vi "main.vi"() -> ()   [LabVIEW 2020]
uses:
  _controls/Notifier Cluster.ctl
  _globals/Global Controls.vi
  <resource>/objmgr/imaqdx.rc
  _controls/Global Ctrl Refs.ctl
  _controls/Trapping Laser Control.ctl
  _controls/Timer_actions.ctl
  <vilib>/userDefined/High Color/IMAQdx.ctl
  _controls/xiCam.ctl
  _controls/PCIe SLM params.ctl
  _controls/Spot Params.ctl
  _controls/PCIe SLM Spots.ctl
  _controls/PCIe SLM Zernike Coefs.ctl
  <vilib>/vision/driver/NI_Vision_Acquisition_Software.lvlib
  _controls/Exp Params.ctl
  _controls/Logging Cluster.ctl
  <vilib>/platform/TimedLoop/XDataNode/XDataNode.xnode
  <vilib>/Platform/TimedLoop/XDataNode/nitl_modes.ctl
  <vilib>/Platform/TimedLoop/XDataNode/XDNodeRunTimeDep.lvlib
  <vilib>/Platform/TimedLoop/XDataNode/wakeup.ctl
  <vilib>/Platform/TimedLoop/XDataNode/timing_clust.ctl
  _controls/SLM Real World to IMAQ Display Transform.ctl
panel:
  out "LIVE":bool
  out "ImgSat":bool
  out "xiCam":T1(plugin-control)
  out "ImgHist":u32[](graph)
  in  "Set ROI":bool
  in  "Reset ROI":bool
  out "fps":dbl caption="Camera Frame Rate (Hz)" format="%0.2f"
  out "SLM Temp (C)":dbl
  out "READY":bool
  in  "LoadXML":bool
  in  "Show Hologram":bool
  in  "SaveCurrentXML":bool
  in  "AcquireSnap":bool
  in  "stop live":bool
  in  "Cam Live Display":bool
  in  "Tab Control":T2(tab)
  in  "Camera Controls":T3={"Exposure Time (ms)"=27, "cam0 Session"="cam0", "Camera ROI"={"Width"=2048, "Height"=2048, "Offset X"=0, "Offset Y"=0}, "Command"=""} {"Camera ROI"."Offset Y" max=2046 step=2; "Camera ROI"."Offset X" max=2044 step=4; "Camera ROI"."Height" min=2 max=2048 step=2; "Camera ROI"."Width" min=4 max=2048 step=4; "Exposure Time (ms)" min=27 max=500 step=1 scale=27.0..500.0}
  in  "Spots":T5={"Spot Params"=[{"Intensity"=1.0, "Vortex"=0.0, "Phase"=0.0, "X"=0.0, "Y"=0.0, "Z"=0.0}], "Add Spot"=FALSE, "Remove Spot"=FALSE, "Clear All Spots"=FALSE, "Save Spots"=FALSE, "Generate Spots"=FALSE, "Generate Spot Pattern"=""} {"Spot Params"."Z" format="%_4g"; "Spot Params"."Y" format="%_4g"; "Spot Params"."X" format="%_4g"; "Spot Params"."Phase" format="%_4g"; "Spot Params"."Intensity" format="%_4g"}
  in  "Ventus Controls":T7 caption="Trapping Laser" {"Ventus Power" min=0.0 max=100.0 step=0.1 scale=0.0..100.0}
  in  "GridSpotsNoiseAmp":dbl=1000.0 caption="Noise Amplitude for 9x9 Grid"
  in  "Grid Size x":i32=10
  in  "Grid Size Y":i32=40
  out "Saving To Disk":i32(slide) scale=-1.0..21600.0
  out "AcqData":i32(slide) max=1000 scale=-1.0..21600.0
  in  "Exp Params":T8={"Experiment Type"="Time Series", "Experiment Name"="Experiment_1", "ExpPath"=path "D:/Data", "Save As"="TIFF", "TSFrames"=1000, "TSfps"=1.0, "Streaming"=TRUE, "tdms ref"=refnum, "frame #"=0, "Full Path"=path "", "PeakOnQueue"=FALSE} {"TSFrames" min=1 step=1; "TSfps" min=0.001 max=90.0 step=0.001 format="%_4g"}
  in  "Start Acquisition":bool
  in  "StopAcq":bool
  in  "SLM to IMAQ":T9={"Translation"={"X"=255.9856, "Y"=245.976}, "Scalling"={"xScale"=2.61758691206544, "yScale"=-2.61759}}
  out "LUT Graph":cluster{"X":dbl, "Y":dbl}[](graph)=[{"X"=-3.141592653589793, "Y"=0.0}, {"X"=-3.1169527112086968, "Y"=0.0}, {"X"=-3.0923127688276004, "Y"=0.0}, {"X"=-3.067672826446504, "Y"=0.0}, {"X"=-3.0430328840654073, "Y"=0.0}, {"X"=-3.018392941684311, "Y"=0.0}, {"X"=-2.9937529993032146, "Y"=0.0}, {"X"=-2.9691130569221182, "Y"=0.004441683995677549}, {"X"=-2.944473114541022, "Y"=0.009393597048351928}, {"X"=-2.9198331721599255, "Y"=0.014387507250025256}, {"X"=-2.8951932297788288, "Y"=0.01942901000939432}, {"X"=-2.8705532873977324, "Y"=0.024523700735155904}, {"X"=-2.845913345016636, "Y"=0.029677174836006792}, {"X"=-2.8212734026355397, "Y"=0.03489502772064378}, {"X"=-2.7966334602544434, "Y"=0.04018285479776366}, {"X"=-2.771993517873347, "Y"=0.045546251476063185}, {"X"=-2.7473535754922507, "Y"=0.050990796622549954}, {"X"=-2.722713633111154, "Y"=0.05651951641111443}, {"X"=-2.6980736907300575, "Y"=0.062130151145079436}, {"X"=-2.673433748348961, "Y"=0.06781978536195998}, {"X"=-2.648793805967865, "Y"=0.07358550359927116}, {"X"=-2.6241538635867685, "Y"=0.07942439039452798}, {"X"=-2.5995139212056717, "Y"=0.0853335302852455}, {"X"=-2.5748739788245754, "Y"=0.09131000780893878}, {"X"=-2.550234036443479, "Y"=0.09735090750312286}, {"X"=-2.5255940940623827, "Y"=0.10345331390531276}, {"X"=-2.5009541516812863, "Y"=0.10961431155302359}, {"X"=-2.47631420930019, "Y"=0.11583098498377034}, {"X"=-2.4516742669190936, "Y"=0.12210041873506809}, {"X"=-2.4270343245379973, "Y"=0.12841969734443184}, {"X"=-2.4023943821569005, "Y"=0.1347859053493767}, {"X"=-2.377754439775804, "Y"=0.14119612728741773}, {"X"=-2.353114497394708, "Y"=0.1476474476960699}, {"X"=-2.3284745550136114, "Y"=0.15413695111284825}, {"X"=-2.303834612632515, "Y"=0.16066172207526794}, {"X"=-2.2791946702514183, "Y"=0.1672188451208439}, {"X"=-2.254554727870322, "Y"=0.17380540478709125}, {"X"=-2.2299147854892256, "Y"=0.18041848561152501}, {"X"=-2.2052748431081293, "Y"=0.1870551721316602}, {"X"=-2.180634900727033, "Y"=0.19371254888501188}, {"X"=-2.1559949583459366, "Y"=0.20038770040909518}, {"X"=-2.1313550159648402, "Y"=0.20707771124142504}, {"X"=-2.106715073583744, "Y"=0.21377966591951653}, {"X"=-2.082075131202647, "Y"=0.22049064898088477}, {"X"=-2.0574351888215507, "Y"=0.22720774496304472}, {"X"=-2.0327952464404544, "Y"=0.23392803840351145}, {"X"=-2.008155304059358, "Y"=0.24064861383980002}, {"X"=-1.9835153616782615, "Y"=0.2473665558094255}, {"X"=-1.9588754192971651, "Y"=0.2540789488499029}, {"X"=-1.9342354769160686, "Y"=0.2607828774987472}, {"X"=-1.9095955345349722, "Y"=0.2674754262934736}, {"X"=-1.8849555921538759, "Y"=0.27415367977159705}, {"X"=-1.8603156497727795, "Y"=0.2808147224706326}, {"X"=-1.835675707391683, "Y"=0.2874556389280954}, {"X"=-1.8110357650105866, "Y"=0.2940735136815004}, {"X"=-1.78639582262949, "Y"=0.3006654312683626}, {"X"=-1.761755880248394, "Y"=0.30722847622619714}, {"X"=-1.7371159378672973, "Y"=0.313759733092519}, {"X"=-1.712475995486201, "Y"=0.32025628640484327}, {"X"=-1.6878360531051044, "Y"=0.326715220700685}, {"X"=-1.663196110724008, "Y"=0.3331336205175592}, {"X"=-1.6385561683429117, "Y"=0.339508570392981}, {"X"=-1.6139162259618154, "Y"=0.34583715486446537}, {"X"=-1.5892762835807188, "Y"=0.3521164584695273}, {"X"=-1.5646363411996225, "Y"=0.35834356574568205}, {"X"=-1.5399963988185261, "Y"=0.36451556123044443}, {"X"=-1.5153564564374296, "Y"=0.37062952946132965}, {"X"=-1.4907165140563332, "Y"=0.3766825549758526}, {"X"=-1.4660765716752369, "Y"=0.38267172231152863}, {"X"=-1.4414366292941405, "Y"=0.3885943072376766}, {"X"=-1.4167966869130437, "Y"=0.3944495212813968}, {"X"=-1.3921567445319474, "Y"=0.40023770070543735}, {"X"=-1.3675168021508513, "Y"=0.40595919565461763}, {"X"=-1.342876859769755, "Y"=0.41161435627375703}, {"X"=-1.3182369173886581, "Y"=0.4172035327076747}, {"X"=-1.2935969750075618, "Y"=0.42272707510119023}, {"X"=-1.2689570326264654, "Y"=0.4281853335991228}, {"X"=-1.244317090245369, "Y"=0.43357865834629183}, {"X"=-1.2196771478642725, "Y"=0.4389073994875166}, {"X"=-1.1950372054831762, "Y"=0.4441719071676165}, {"X"=-1.1703972631020798, "Y"=0.4493725315314109}, {"X"=-1.1457573207209835, "Y"=0.4545096227237191}, {"X"=-1.121117378339887, "Y"=0.45958353088936044}, {"X"=-1.0964774359587905, "Y"=0.4645946061731544}, {"X"=-1.0718374935776942, "Y"=0.4695431987199201}, {"X"=-1.0471975511965979, "Y"=0.474429658674477}, {"X"=-1.022557608815501, "Y"=0.4792543361816445}, {"X"=-0.9979176664344047, "Y"=0.48401758138624185}, {"X"=-0.9732777240533084, "Y"=0.4887197444330884}, {"X"=-0.948637781672212, "Y"=0.49336117546700364}, {"X"=-0.9239978392911157, "Y"=0.49794222463280674}, {"X"=-0.8993578969100193, "Y"=0.502463242075317}, {"X"=-0.874717954528923, "Y"=0.5069245779393541}, {"X"=-0.8500780121478266, "Y"=0.511326582369737}, {"X"=-0.8254380697667298, "Y"=0.5156696055112853}, {"X"=-0.8007981273856335, "Y"=0.5199539975088181}, {"X"=-0.7761581850045371, "Y"=0.5241801085071551}, {"X"=-0.7515182426234408, "Y"=0.5283482886511154}, {"X"=-0.726878300242344, "Y"=0.5324588880855183}, {"X"=-0.7022383578612477, "Y"=0.5365122569551832}, {"X"=-0.6775984154801513, "Y"=0.5405087454049295}, {"X"=-0.652958473099055, "Y"=0.5444487035795768}, {"X"=-0.6283185307179586, "Y"=0.5483324816239438}, {"X"=-0.6036785883368623, "Y"=0.5521604296828504}, {"X"=-0.5790386459557659, "Y"=0.5559328979011158}, {"X"=-0.5543987035746696, "Y"=0.5596502364235592}, {"X"=-0.5297587611935728, "Y"=0.563312795395}, {"X"=-0.5051188188124764, "Y"=0.5669209249602577}, {"X"=-0.4804788764313801, "Y"=0.5704749752641516}, {"X"=-0.45583893405028375, "Y"=0.5739752964515009}, {"X"=-0.43119899166918696, "Y"=0.5774222386671249}, {"X"=-0.4065590492880906, "Y"=0.5808161520558432}, {"X"=-0.3819191069069947, "Y"=0.5841573867624752}, {"X"=-0.35727916452589836, "Y"=0.5874462929318399}, {"X"=-0.33263922214480157, "Y"=0.5906832207087569}, {"X"=-0.3079992797637052, "Y"=0.5938685202380454}, {"X"=-0.2833593373826089, "Y"=0.5970025416645248}, {"X"=-0.25871939500151253, "Y"=0.6000856351330144}, {"X"=-0.23407945262041574, "Y"=0.6031181507883338}, {"X"=-0.2094395102393194, "Y"=0.606100438775302}, {"X"=-0.18479956785822305, "Y"=0.6090328492387385}, {"X"=-0.1601596254771267, "Y"=0.6119157323234626}, {"X"=-0.13551968309603035, "Y"=0.6147494381742937}, {"X"=-0.110879740714934, "Y"=0.6175343169360511}, {"X"=-0.08623979833383766, "Y"=0.6202707187535542}, {"X"=-0.06159985595274131, "Y"=0.6229589937716223}, {"X"=-0.03695991357164452, "Y"=0.6255994921350748}, {"X"=-0.012319971190548173, "Y"=0.628192563988731}, {"X"=0.012319971190548173, "Y"=0.6307385594774102}, {"X"=0.03695991357164452, "Y"=0.6332378287459319}, {"X"=0.06159985595274087, "Y"=0.6356907219391152}, {"X"=0.08623979833383721, "Y"=0.6380975892017797}, {"X"=0.110879740714934, "Y"=0.6404587806787446}, {"X"=0.13551968309603035, "Y"=0.6427746465148293}, {"X"=0.1601596254771267, "Y"=0.6450455368548531}, {"X"=0.18479956785822305, "Y"=0.6472718018436354}, {"X"=0.2094395102393194, "Y"=0.6494537916259955}, {"X"=0.23407945262041574, "Y"=0.6515918563467528}, {"X"=0.2587193950015121, "Y"=0.6536863461507265}, {"X"=0.28335933738260843, "Y"=0.6557376111827362}, {"X"=0.30799927976370567, "Y"=0.657746001587601}, {"X"=0.332639222144802, "Y"=0.6597118675101404}, {"X"=0.35727916452589836, "Y"=0.6616355590951737}, {"X"=0.3819191069069947, "Y"=0.6635174264875202}, {"X"=0.4065590492880906, "Y"=0.6653578198319992}, {"X"=0.43119899166918696, "Y"=0.6671570892734301}, {"X"=0.4558389340502833, "Y"=0.6689155849566324}, {"X"=0.48047887643137965, "Y"=0.6706336570264253}, {"X"=0.5051188188124769, "Y"=0.6723116556276281}, {"X"=0.5297587611935732, "Y"=0.6739499309050603}, {"X"=0.5543987035746696, "Y"=0.6755488330035411}, {"X"=0.5790386459557659, "Y"=0.6771087120678899}, {"X"=0.6036785883368623, "Y"=0.6786299182429261}, {"X"=0.6283185307179586, "Y"=0.6801128016734688}, {"X"=0.652958473099055, "Y"=0.6815577125043376}, {"X"=0.6775984154801513, "Y"=0.6829650008803521}, {"X"=0.7022383578612481, "Y"=0.6843350169463309}, {"X"=0.7268783002423445, "Y"=0.6856681108470939}, {"X"=0.7515182426234408, "Y"=0.6869646327274603}, {"X"=0.7761581850045371, "Y"=0.6882249327322496}, {"X"=0.8007981273856335, "Y"=0.6894493610062808}, {"X"=0.8254380697667298, "Y"=0.6906382676943738}, {"X"=0.8500780121478262, "Y"=0.6917920029413474}, {"X"=0.8747179545289221, "Y"=0.6929109168920209}, {"X"=0.8993578969100193, "Y"=0.6939953596912143}, {"X"=0.9239978392911157, "Y"=0.6950456814837462}, {"X"=0.948637781672212, "Y"=0.6960622324144364}, {"X"=0.9732777240533084, "Y"=0.6970453626281042}, {"X"=0.9979176664344047, "Y"=0.6979954222695688}, {"X"=1.022557608815501, "Y"=0.6989127614836497}, {"X"=1.0471975511965974, "Y"=0.699797730415166}, {"X"=1.0718374935776938, "Y"=0.7006506792089373}, {"X"=1.096477435958791, "Y"=0.7014719880473896}, {"X"=1.1211173783398873, "Y"=0.7022625378987619}, {"X"=1.1457573207209837, "Y"=0.703023623303892}, {"X"=1.17039726310208, "Y"=0.7037565511981412}, {"X"=1.1950372054831764, "Y"=0.7044626285168711}, {"X"=1.2196771478642727, "Y"=0.7051431621954433}, {"X"=1.244317090245369, "Y"=0.7057994591692192}, {"X"=1.2689570326264654, "Y"=0.7064328263735603}, {"X"=1.2935969750075618, "Y"=0.7070445707438283}, {"X"=1.3182369173886581, "Y"=0.7076359992153846}, {"X"=1.3428768597697545, "Y"=0.7082084187235906}, {"X"=1.3675168021508508, "Y"=0.7087631362038079}, {"X"=1.3921567445319472, "Y"=0.7093014585913984}, {"X"=1.4167966869130435, "Y"=0.7098246928217231}, {"X"=1.4414366292941398, "Y"=0.7103341458301439}, {"X"=1.4660765716752362, "Y"=0.7108311245520219}, {"X"=1.4907165140563334, "Y"=0.7113169359227188}, {"X"=1.5153564564374298, "Y"=0.7117928868775963}, {"X"=1.5399963988185261, "Y"=0.7122602843520158}, {"X"=1.5646363411996225, "Y"=0.7127204352813389}, {"X"=1.5892762835807188, "Y"=0.713174646600927}, {"X"=1.6139162259618152, "Y"=0.7136242252461416}, {"X"=1.6385561683429115, "Y"=0.7140704781523443}, {"X"=1.6631961107240079, "Y"=0.7145147122548965}, {"X"=1.687836053105105, "Y"=0.71495823448916}, {"X"=1.7124759954862014, "Y"=0.7154023517904959}, {"X"=1.7371159378672978, "Y"=0.7158483710942662}, {"X"=1.7617558802483941, "Y"=0.7162975993358321}, {"X"=1.7863958226294905, "Y"=0.7167513434505554}, {"X"=1.8110357650105868, "Y"=0.717210910373797}, {"X"=1.8356757073916832, "Y"=0.7176776070409191}, {"X"=1.8603156497727795, "Y"=0.718152740387283}, {"X"=1.8849555921538759, "Y"=0.7186376173482502}, {"X"=1.9095955345349722, "Y"=0.7191335448591821}, {"X"=1.9342354769160686, "Y"=0.7196418298554405}, {"X"=1.958875419297165, "Y"=0.7201637792723864}, {"X"=1.9835153616782613, "Y"=0.7207007000453821}, {"X"=2.0081553040593576, "Y"=0.7212538991097884}, {"X"=2.032795246440454, "Y"=0.7218246834009672}, {"X"=2.0574351888215503, "Y"=0.7224143598542799}, {"X"=2.0820751312026475, "Y"=0.7230242354050881}, {"X"=2.106715073583744, "Y"=0.7236556169887532}, {"X"=2.1313550159648402, "Y"=0.724309811540637}, {"X"=2.1559949583459366, "Y"=0.7249881259961006}, {"X"=2.180634900727033, "Y"=0.7256918672905059}, {"X"=2.2052748431081293, "Y"=0.726422342359214}, {"X"=2.2299147854892256, "Y"=0.727180858137587}, {"X"=2.254554727870322, "Y"=0.7279687215609859}, {"X"=2.279194670251419, "Y"=0.7287872395647725}, {"X"=2.3038346126325155, "Y"=0.7296377190843082}, {"X"=2.328474555013612, "Y"=0.7305214670549545}, {"X"=2.3531144973947082, "Y"=0.7314397904120732}, {"X"=2.3777544397758037, "Y"=0.7323939960910253}, {"X"=2.4023943821569, "Y"=0.7333853910271728}, {"X"=2.4270343245379964, "Y"=0.734415282155877}, {"X"=2.4516742669190927, "Y"=0.7354849764124994}, {"X"=2.47631420930019, "Y"=0.7365957807324018}, {"X"=2.5009541516812863, "Y"=0.7377490020509453}, {"X"=2.5255940940623827, "Y"=0.7389459473034917}, {"X"=2.550234036443479, "Y"=0.7401879234254024}, {"X"=2.5748739788245754, "Y"=0.7414762373520393}, {"X"=2.5995139212056717, "Y"=0.7428121960187631}, {"X"=2.624153863586768, "Y"=0.7441971063609361}, {"X"=2.6487938059678644, "Y"=0.7456322753139194}, {"X"=2.6734337483489616, "Y"=0.7471192148964195}, {"X"=2.698073690730058, "Y"=0.7486625931433437}, {"X"=2.7227136331111543, "Y"=0.7502695530679421}, {"X"=2.7473535754922507, "Y"=0.751947304031351}, {"X"=2.771993517873347, "Y"=0.7537030553947075}, {"X"=2.7966334602544434, "Y"=0.7555440165191485}, {"X"=2.8212734026355397, "Y"=0.7574773967658104}, {"X"=2.845913345016636, "Y"=0.7595104054958302}, {"X"=2.8705532873977324, "Y"=0.7616502520703445}, {"X"=2.8951932297788288, "Y"=0.7639041458504902}, {"X"=2.919833172159925, "Y"=0.7662792961974041}, {"X"=2.9444731145410215, "Y"=0.7687829124722226}, {"X"=2.969113056922118, "Y"=0.7714222040360831}, {"X"=2.993752999303214, "Y"=0.7742043802501217}, {"X"=3.0183929416843105, "Y"=0.7771366504754755}, {"X"=3.043032884065407, "Y"=0.7802262240732813}, {"X"=3.067672826446504, "Y"=0.7834803104046757}, {"X"=3.0923127688276004, "Y"=0.7869061188307955}, {"X"=3.1169527112086968, "Y"=0.7905108587127776}, {"X"=3.141592653589793, "Y"=0.7943017394117585}]
  in  "Zernikes":T10 caption="Zernike Coefficients" {"SecComaY" step=0.01; "SecComaX" step=0.01; "SecAstigY" step=0.01; "SecAstigX" step=0.01; "ComaY" step=0.01; "ComaX" step=0.01; "AstigY" step=0.01; "AstigX" step=0.01}
  in  "SLM Parameters":T11={"Width"=1920.0, "Height"=1152.0, "Board ID"=1, "Centre Y"=0.46199999999999997, "Centre X"=0.3859999999999999} {"Centre X" format="%.3g"; "Centre Y" format="%.3g"}
  in  "Master Stop":bool
  # "Notes\n\nAs of Oct 2024\n\nNon-Streaming acquisition is now controlled with the Frame Rate (Hz) control.\n\nThe slowest acquisition is 1 Hz. This is due to the limitiations of the cameras driver.\n\nPeaking during acquisition will show a real time image. Do not use in the case of high speed acquisitions as this may slow things down.\n\nSnapshots are fixed.\n\nSaving as TDMS works but is a little slower than saving as TIFF. Still advisable, since you end up with one file regardless of acquisition size."
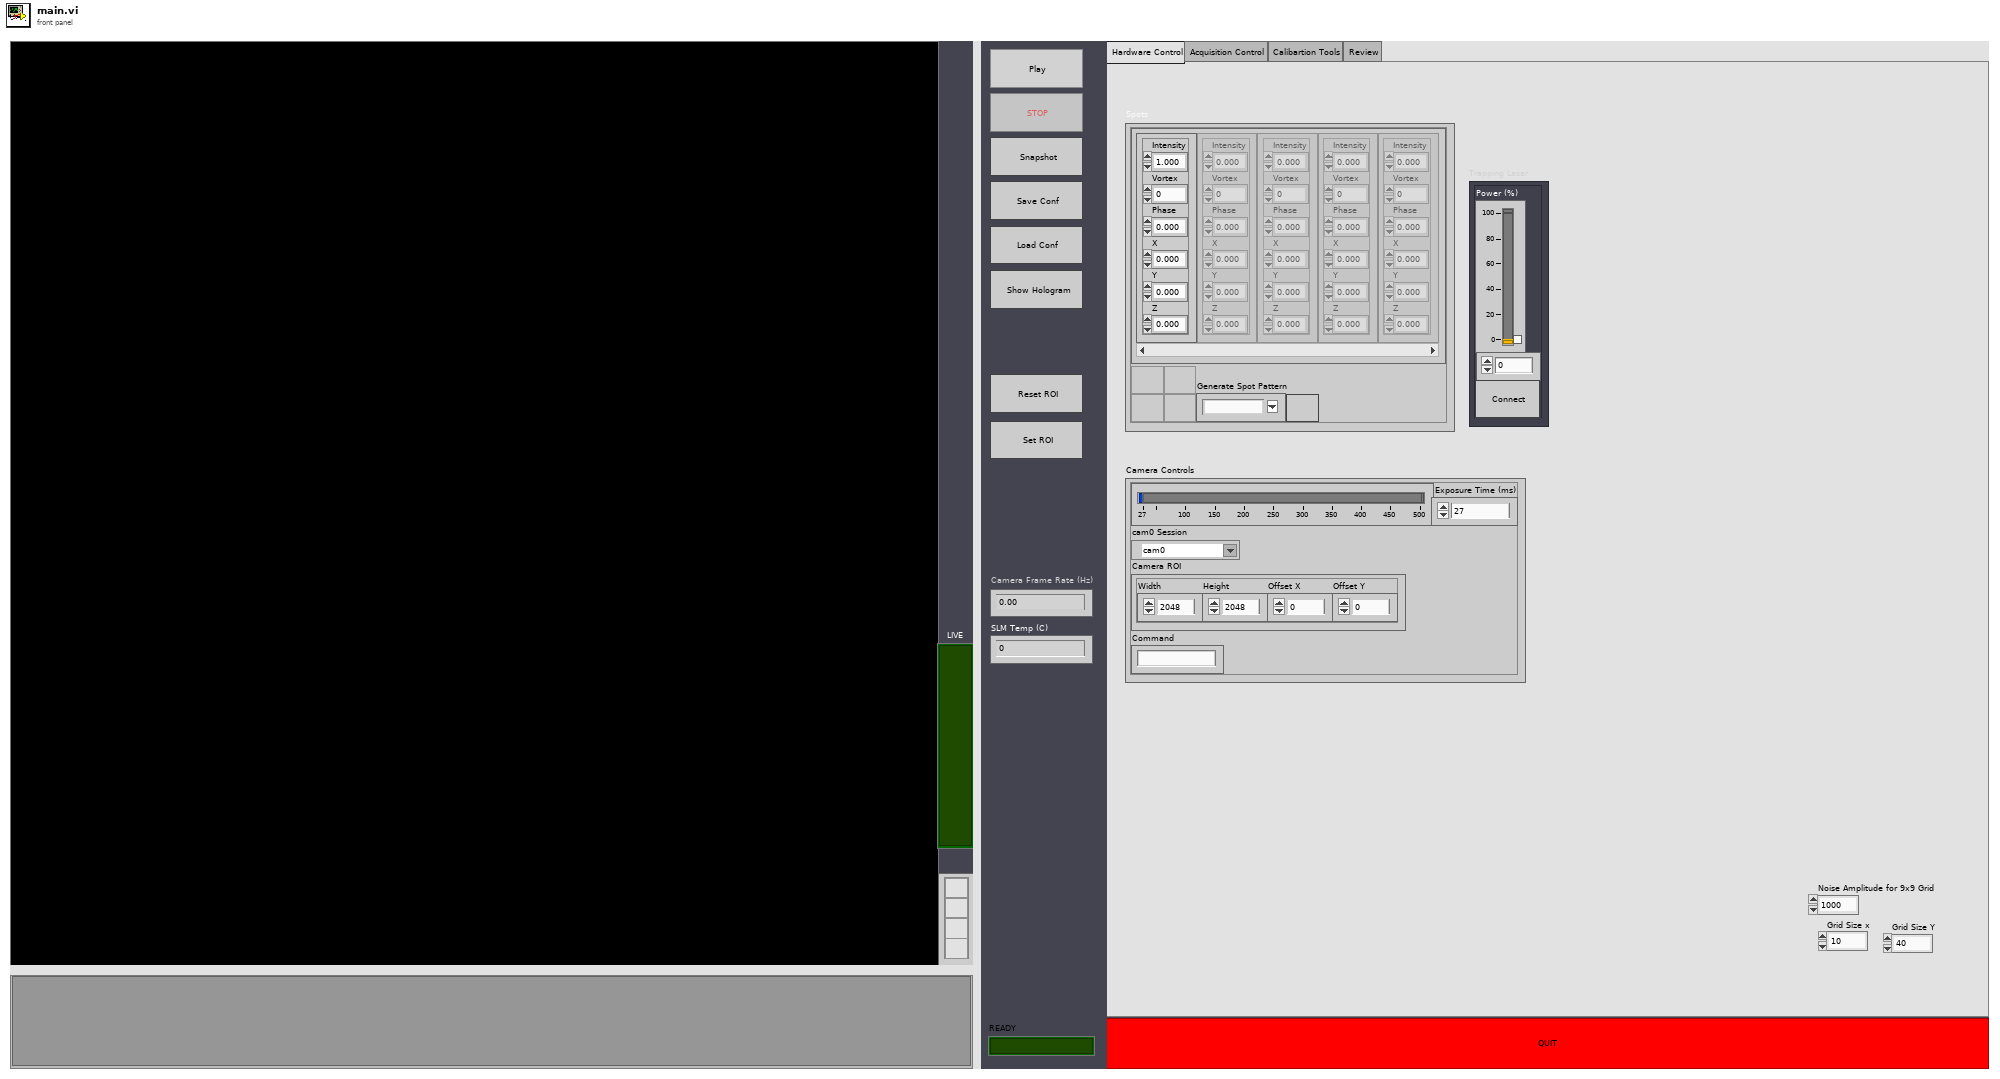
[diagram p1: front panel]
types:
  T1 = typedef "IMAQ Image.ctl" = refnum<image>
  T2 = enum32{"Hardware Control", "Acquisition Control", "Calibartion Tools", "Review"}
  T3 = typedef "xiCam.ctl" = cluster{"Exposure Time (ms)":u32, "cam0 Session":T4, "Camera ROI":cluster{"Width":u32, "Height":u32, "Offset X":u32, "Offset Y":u32}, "Command":string}
  T4 = typedef "IMAQdx.ctl" = refnum<k21>
  T5 = typedef "PCIe SLM Spots.ctl" = cluster{"Spot Params":T6, "Add Spot":bool, "Remove Spot":bool, "Clear All Spots":bool, "Save Spots":bool, "Generate Spots":bool, "Generate Spot Pattern":string}
  T6 = typedef "Spot Params.ctl" = cluster{"Intensity":dbl, "Vortex":dbl, "Phase":dbl, "X":dbl, "Y":dbl, "Z":dbl}[]
  T7 = typedef "Trapping Laser Control.ctl" = cluster{"Ventus Power":dbl, "Open Serial":bool, "VISA Refnum":refnum<visa-resource-name>}
  T8 = typedef "Exp Params.ctl" = cluster{"Experiment Type":string, "Experiment Name":string, "ExpPath":path, "Save As":string, "TSFrames":i32, "TSfps":dbl, "Streaming":bool, "tdms ref":refnum<k34>, "frame #":i64, "Full Path":path, "PeakOnQueue":bool}
  T9 = typedef "SLM Real World to IMAQ Display Transform.ctl" = cluster{"Translation":cluster{"X":dbl, "Y":dbl}, "Scalling":cluster{"xScale":dbl, "yScale":dbl}}
  T10 = typedef "PCIe SLM Zernike Coefs.ctl" = cluster{"enabled":bool, "AstigX":dbl, "AstigY":dbl, "ComaX":dbl, "ComaY":dbl, "SecAstigX":dbl, "SecAstigY":dbl, "SecComaX":dbl, "SecComaY":dbl}
  T11 = typedef "PCIe SLM params.ctl" = cluster{"Width":dbl, "Height":dbl, "Board ID":i32, "Centre Y":dbl, "Centre X":dbl}
  T12 = enum8{"Enabled", "Disabled", "Disabled and Grayed Out"}
  T13 = typedef "Image Type" = u32
  T14 = typedef "Global Ctrl Refs.ctl" = cluster{"Exp Params":refnum<vi>, "Ventus Controls":refnum<vi>, "SLM Parameters":refnum<vi>, "Spot Params":refnum<vi>, "Camera Controls":refnum<vi>}
  T15 = typedef "Global Ctrls For Saving.ctl" = cluster{"Time Stamp":cluster{"date string":string, "time string":string}, "Exp Params":T8, "Ventus Controls":T7, "Camera Controls":T3, "Spot Params":T6, "SLM Parameters":T11}
  T16 = typedef "Notifiers.ctl" = cluster{"Instrument Control":refnum<notifier>, "Live Display":refnum<notifier>, "Acquisition":refnum<notifier>}
  T17 = typedef "XDNodeRunTimeDep.lvlib/timing_clust.ctl" = cluster{"Expected End [f-1]":u64, "Actual End [f-1]":u64, "Finished Late? [f-1]":bool, "Expected End [i-1]":u64, "Actual End [i-1]":u64, "Finished Late? [i-1]":bool, "Expected Start [i]":u64, "Actual Start [i]":u64, "Expected Start [f]":u64, "Actual Start [f]":u64, "Source Name":string, "Structure Name":string, "Period":i64, "Deadline":i64, "Offset":i64, "Start":i64, "Priority":i32, "Timeout":i32, "Mode":T18, "Wakeup Reason":T19, "Error":errorcluster, "Source Type":string, "Secondary Source Type":string, "Global End Time":u64, "Global Start Time":u64, "Frame Duration":u64, "Iteration Duration":u64, "Assigned CPU":i32, "I/O Scan Engine Mode":u32}
  T18 = typedef "XDNodeRunTimeDep.lvlib/nitl_modes.ctl" = enum32{"No Change", "Process missed periods, maintain original phase", "Discard missed periods, maintain original phase", "Process missed periods, ignore original phase", "Discard missed periods, ignore original phase"}
  T19 = typedef "XDNodeRunTimeDep.lvlib/wakeup.ctl" = enum32{"Normal", "Aborted", "Asynchronous wakeup", "Timing source error", "Timed loop error", "Timeout"}
  T20 = typedef "Logging Cluster.ctl" = cluster{"Image Data Array":u8[], "Buffer Number":i32, "Timestamp (um)":u64, "Exp params":T8}
  T21 = typedef "Timer_actions.ctl" = enum16{"Reset", "Snap", "Total"}
  T22 = cluster{"Width":u32, "Height":u32, "Offset X":u32, "Offset Y":u32}
  T23 = cluster{"Exposure Time (ms)":bool, "cam0 Session":bool, "Camera ROI":cluster{"Width":bool, "Height":bool, "Offset X":bool, "Offset Y":bool}, "Command":bool}
  T24 = cluster{"Global Rectangle":i32[], "Contours":cluster{"Contour Type":u32, "ROI Type":u32, "Points":i32[]}[]}
  T25 = cluster{"Spots":T5, "SLM Parameters":T11, "Zernikes":T10}
  T26 = typedef "LVCursorListTypeDef.ctl" = cluster{"Name":string, "Color":u32, "Style":u8, "Point Style":u8, "Name Visible":bool, "Allow Drag":bool, "Cursor Mode":u32, "Plot":i32, "Index":i32, "Position":cluster{"X":dbl, "Y":dbl}, "X Scale":u32, "Y Scale":u32, "Watch Plots":i32[], "Watch All Plots":bool, "Plot Area":i32, "Label Offset":cluster{"X":dbl, "Y":dbl}}[]
  T27 = typedef "Notifier Cluster.ctl" = cluster{"message":string, "data":variant}
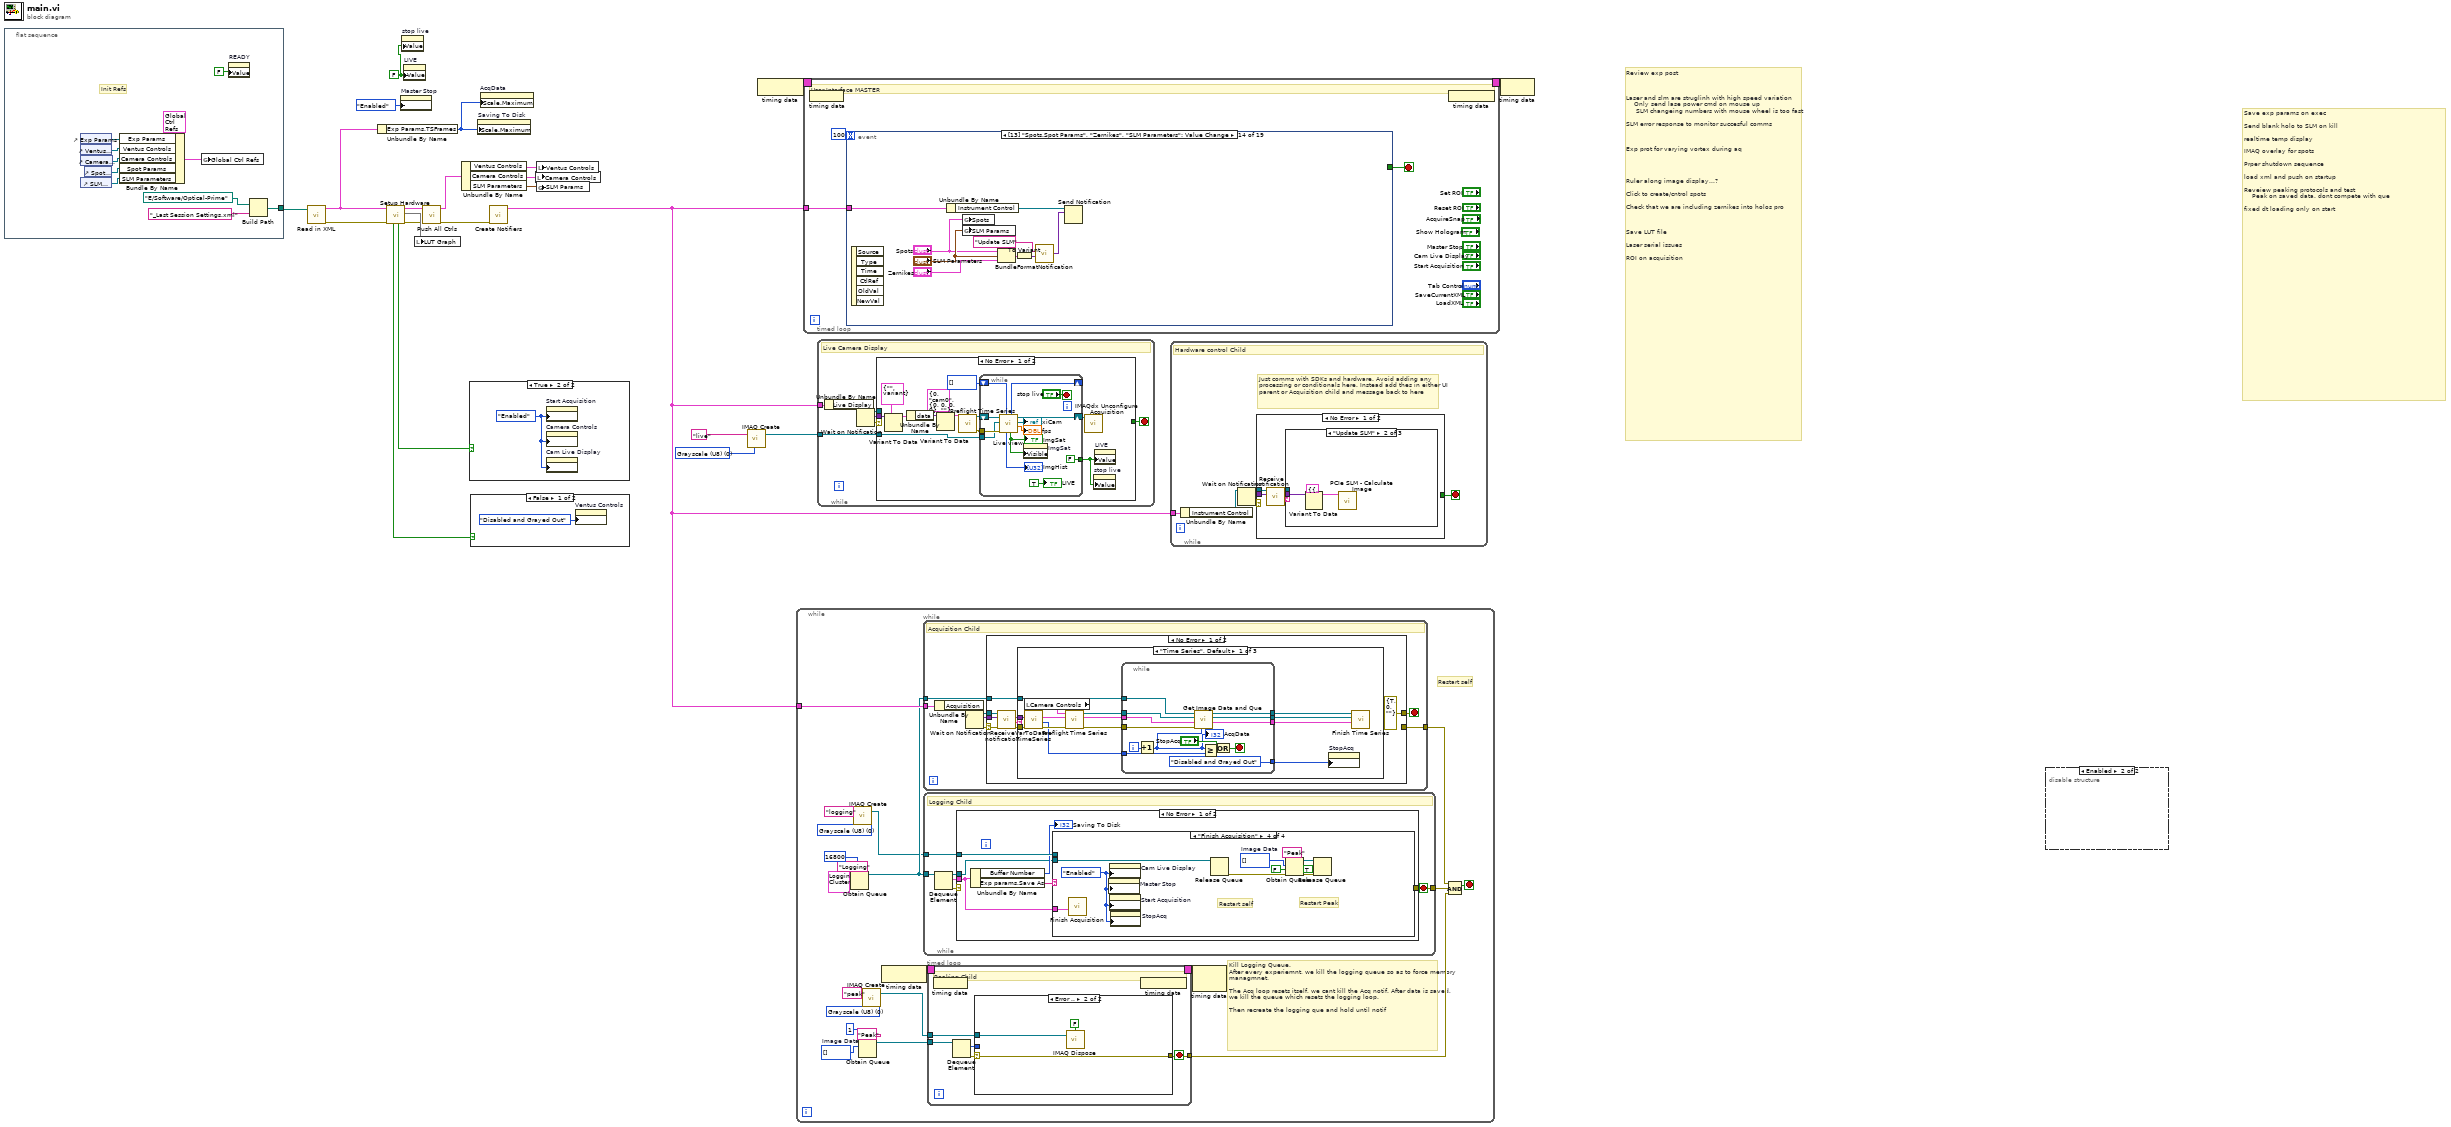
[diagram p0: block diagram]
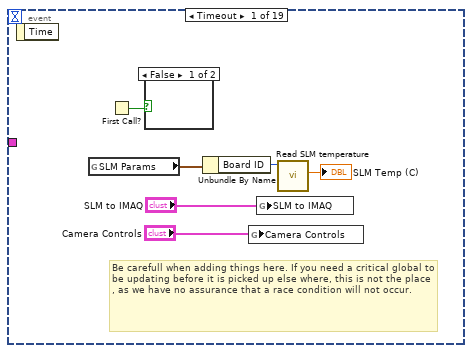
[diagram p2: hidden frame]
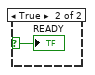
[diagram p3: hidden frame]
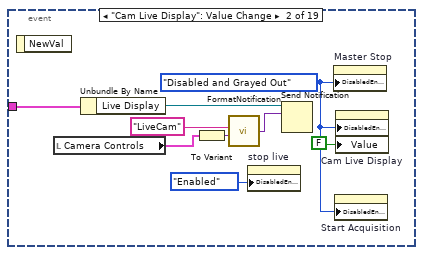
[diagram p4: hidden frame]
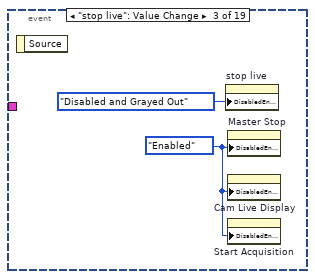
[diagram p5: hidden frame]
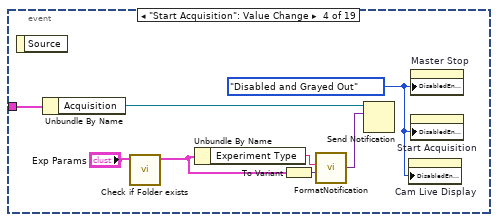
[diagram p6: hidden frame]
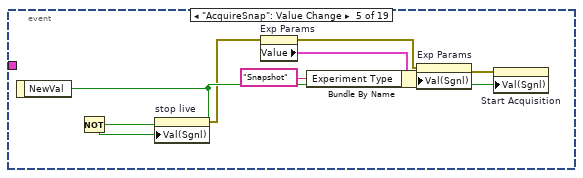
[diagram p7: hidden frame]
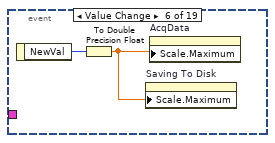
[diagram p8: hidden frame]
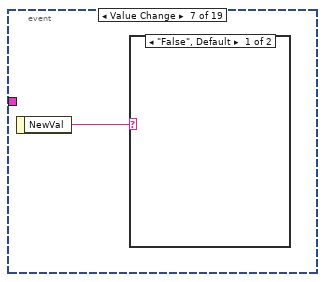
[diagram p9: hidden frame]
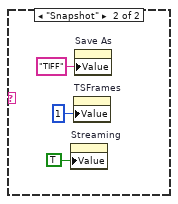
[diagram p10: hidden frame]
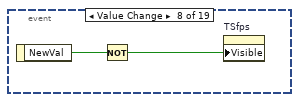
[diagram p11: hidden frame]
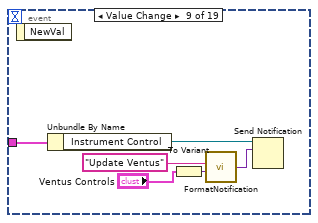
[diagram p12: hidden frame]
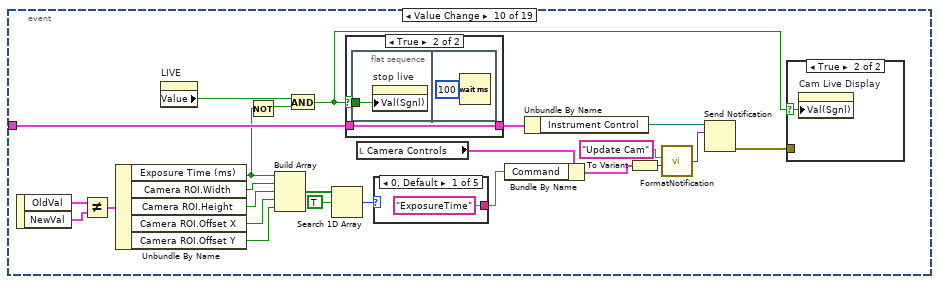
[diagram p13: hidden frame]
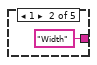
[diagram p16: hidden frame]
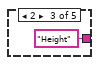
[diagram p17: hidden frame]
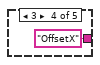
[diagram p18: hidden frame]
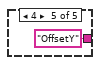
[diagram p19: hidden frame]
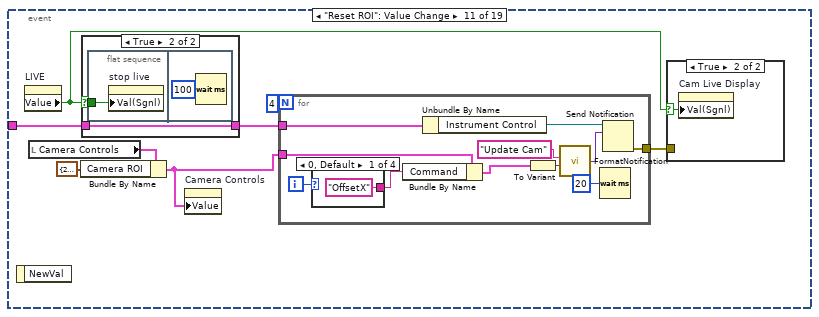
[diagram p20: hidden frame]
diagram:
  w1 = FALSE ("LIVE")
  w22 = T13 0 items=["Grayscale (U8)", "Grayscale (I16)", "Grayscale (SGL)", "Complex (CSG)", "RGB (U32)", "HSL (U32)", "RGB (U64)", "Grayscale (U16)"] ("Image Type")
  # "Save exp params on exec\n\nSend blank holo to SLM on kill\n\nrealtime temp display\n\nIMAQ overlay for spots\n\nPrper shutdown sequence\n\nload xml and push on startup\n\nReveiew peaking protocols and test\n    Peak on saved data. dont compete with que\n\nfixed dt loading only on start"
  # "Review exp post\n\n\n\nLaser and slm are struglinh with high speed variation\n    Only send lase power cmd on mouse up\n     SLM changeing numbers with mouse wheel is too fast\n\nSLM error response to monitor succesful comms\n\n\n\nExp prot for varying vortex during aq\n\n\n\n\nRuler along image display...?\n\nClick to create/cntrol spots\n\nCheck that we are including zernikes into holos pro\n\n\n\nSave LUT file\n\nLaser serial issues\n\nROI on acquisition"
  n1 = flat-sequence {
    tunnel: [w30] -> w5
    frame #0 {
      # "Init Refs"
      n2 = control-ref of="Exp Params"() -> (w27:refnum<vi>)
      n3 = control-ref of="Ventus Controls"() -> (w26:refnum<vi>)
      n4 = control-ref of="SLM Parameters"() -> (w33:refnum<vi>)
      n5 = control-ref of="Camera Controls"() -> (w23:refnum<vi>)
      n6 = control-ref of="Spot Params"() -> (w25:refnum<vi>)
      n7 = Bundle By Name(cluster=T14 {"Exp Params"=refnum, "Ventus Controls"=refnum, "SLM Parameters"=refnum, "Spot Params"=refnum, "Camera Controls"=refnum} ("Optical Prime Controls For Saving"), "Exp Params"=w27, "Ventus Controls"=w26, "Camera Controls"=w23, "Spot Params"=w25, "SLM Parameters"=w33) -> (w29:T14)
      n8 = global write "Global Controls.vi" "Global Ctrl Refs"(w29) -> ()
      n9 = property on="READY" class="Bool (strict)"("Value"=FALSE ("Boolean")) -> ()  [unwired: 2 in, 2 out]
      n10 = Build Path(base path=path "E:/Software/Optical-Prime" ("path"), name or relative path="_Last Session Settings.xml") -> (appended path=w30:path)
    }
  }
  n11 = call "Read in XML.vi"("Path to XML"=w5) -> ("error out"=w13:errorcluster, "OpticalPrime Ctrls For Saving"=w14:T15)  [unwired: 9 in]
  n12 = Unbundle By Name(w14) -> ("Exp Params.TSFrames"=w15:i32)
  n13 = call "Setup Hardware.vi"("error in (no error)"=w13, "Global Ctrls For Saving"=w14) -> ("error out"=w10:errorcluster, 2:w11, "Global Ctrls For Saving out"=w12:T15, "Camera Connected"=w17:bool, "Trapping Laser Connected"=w18:bool)  [unwired: 5 in]
  n14 = property on="Master Stop" class="Bool (strict)"("DisabledEnum"=T12."Enabled" ("Disabled")) -> ()  [unwired: 2 in, 2 out]
  n15 = property on="stop live" class="Bool (strict)"("Value"=w1) -> ()  [unwired: 2 in, 2 out]
  n16 = property on="LIVE" class="Bool (strict)"("Value"=w1) -> ()  [unwired: 2 in, 2 out]
  n17 = local write "LUT Graph"(w11) -> ()
  n18 = call "Push All Ctrls.vi"("error in"=w10, "OpticalPrime Ctrls For Saving"=w12) -> ("error out"=w7:errorcluster, "OpticalPrime Ctrls For Saving out"=w9:T15)  [unwired: 8 in]
  n19 = Unbundle By Name(w9) -> ("Ventus Controls"=w8:T7, "Camera Controls"=w4:T3, "SLM Parameters"=w6:T11)
  n20 = case shown="True" w17 {
    frame False {
      w34 = T12."Disabled and Grayed Out" ("Disabled")
      n21 = property on="Start Acquisition" class="Bool"("DisabledEnum"=w34) -> ()  [unwired: 2 in, 2 out]
      n22 = property on="Camera Controls" class="Clust (strict)"("DisabledEnum"=w34) -> ()  [unwired: 2 in, 2 out]
      n23 = property on="Cam Live Display" class="Bool (strict)"("DisabledEnum"=w34) -> ()  [unwired: 2 in, 2 out]
    }
    frame True {
      w35 = T12."Enabled" ("Disabled")
      n24 = property on="Start Acquisition" class="Bool"("DisabledEnum"=w35) -> ()  [unwired: 2 in, 2 out]
      n25 = property on="Camera Controls" class="Clust (strict)"("DisabledEnum"=w35) -> ()  [unwired: 2 in, 2 out]
      n26 = property on="Cam Live Display" class="Bool (strict)"("DisabledEnum"=w35) -> ()  [unwired: 2 in, 2 out]
    }
  }
  n27 = case shown="False" w18 {
    frame False {
      n28 = property on="Ventus Controls" class="Clust (strict)"("DisabledEnum"=T12."Disabled and Grayed Out" ("Disabled")) -> ()  [unwired: 2 in, 2 out]
    }
    frame True {
      n29 = property on="Ventus Controls" class="Clust (strict)"("DisabledEnum"=T12."Enabled" ("Disabled")) -> ()  [unwired: 2 in, 2 out]
    }
  }
  n30 = property on="Saving To Disk" class="Slide (strict)"("Scale.Maximum"=w15) -> ()  [unwired: 2 in, 2 out]
  n31 = property on="AcqData" class="Slide (strict)"("Scale.Maximum"=w15) -> ()  [unwired: 2 in, 2 out]
  n32 = call "Create Notifiers.vi"("error in (no error)"=w7) -> ("notifiers cluster"=w16:T16)  [unwired: 8 in, 2 out]
  n33 = local write "Camera Controls"(w4) -> ()
  n34 = local write "Ventus Controls"(w8) -> ()
  n35 = global write "Global Controls.vi" "SLM Params"(w6) -> ()
  n36 = call "IMAQ Create"("Image Name"="live", "Image Type"=w22) -> ("New Image"=w20:T1)  [unwired: 3 in, 1 out]
  n37 = node-c288() -> (w3:T17)
  n38 = while {
    tunnel: w16 -> [w56]
    stop <- w50 stop-if-true
    (unwired) T13 0 items=["Grayscale (U8)", "Grayscale (I16)", "Grayscale (SGL)", "Complex (CSG)", "RGB (U32)", "HSL (U32)", "RGB (U64)", "Grayscale (U16)"] ("Image Type")
    w43 = u8[] []  # Image Data
    (unwired) T13 0 items=["Grayscale (U8)", "Grayscale (I16)", "Grayscale (SGL)", "Complex (CSG)", "RGB (U32)", "HSL (U32)", "RGB (U64)", "Grayscale (U16)"] ("Image Type")
    # "Kill Logging Queue.\nAfter every experiemnt, we kill the logging queue so as to force memory managmnet.\n\nThe Acq loop resets itself, we cant kill the Acq notif. After data is saved, we kill the queue which resets the logging loop.\n\nThen recreate the logging que and hold until notif"
    # "Restart self"
    n39 = Obtain Queue(max queue size (-1, unlimited)=16800, name (unnamed)="Logging", element data type=T20 {"Image Data Array"=[], "Buffer Number"=0, "Timestamp (um)"=0, "Exp params"={"Experiment Type"="", "Experiment Name"="Experiment_1", "ExpPath"=path "D:/Data", "Save As"="TIFF", "TSFrames"=1000, "TSfps"=1.0, "Streaming"=FALSE, "tdms ref"=refnum, "frame #"=0, "Full Path"=path "", "PeakOnQueue"=FALSE}}) -> (queue out=w53:refnum<queue>)  [unwired: 2 in, 2 out]
    n40 = call "IMAQ Create"("Image Name"="logging") -> ("New Image"=w51:T1)  [unwired: 4 in, 1 out]
    n41 = Obtain Queue(max queue size (-1, unlimited)=1, name (unnamed)="Peak", element data type=w43) -> (queue out=w44:refnum<queue>)  [unwired: 2 in, 2 out]
    n42 = call "IMAQ Create"("Image Name"="peak") -> ("New Image"=w41:T1)  [unwired: 4 in, 1 out]
    n43 = node-c288() -> (w39:T17)
    n44 = while {
      tunnel: w56 -> [w110]
      tunnel: w53 -> [w105]
      tunnel: [w103] -> w48
      stop <- w104 stop-if-true
      # "Acquisition Child"
      n45 = Unbundle By Name(w110) -> ("Acquisition"=w109:refnum<notifier>)
      n46 = Wait on Notification(notifier=w109) -> (notifier out=w107:refnum<notifier>, notification=w106:variant, error out=w108:errorcluster)  [unwired: 3 in, 1 out]
      n47 = case shown="No Error" w108 {
        selector: w108 -> [w113 w165]
        tunnel: [errorcluster {"status"=TRUE, "code"=0, "source"=""} ("error IO") w165] -> w104
        tunnel: w105 -> [w115 w166]
        tunnel: w107 -> [w117 _]
        tunnel: w106 -> [w116 _]
        tunnel: [_ w165] -> w103
        frame No Error {
          n48 = call "Receive notification.vi"("error in"=w113, "Variant"=w116, "notifier in"=w117) -> ("error out"=w112:errorcluster, "message"=w114:string, "data"=w118:variant)  [unwired: 5 in, 1 out]
          n49 = case shown="\"Time Series\", Default" w114 {
            tunnel: w118 -> [w132 w160 _]
            tunnel: w115 -> [w131 w159 _]
            tunnel: w112 -> [w127 w155 _]
            frame "Time Series", Default {
              n50 = local read "Camera Controls"() -> (w128:T3)
              n51 = call "VarToData - TimeSeries.vi"("error in"=w127, "data"=w132) -> ("error out"=w126:errorcluster, "TSFrames"=w125:i32, "Exp params"=w120:T8)  [unwired: 3 in]
              n52 = call "Preflight Time Series.vi"("error in"=w126, "Exp params"=w120, "Camera Controls"=w128) -> ("error out"=w129:errorcluster, "Exp params out"=w119:T8, "CamSession out"=w130:T4)  [unwired: 6 in]
              n53 = while {
                tunnel: w129 -> [w144]
                tunnel: w125 -> [w142]
                tunnel: w119 -> [w135]
                tunnel: [w136] -> w123
                tunnel: [T12."Disabled and Grayed Out" ("Disabled")] -> w122
                tunnel: w130 -> [w146]
                tunnel: [w133] -> w121
                tunnel: w131 -> [w145]
                tunnel: [w139] -> w124
                i -> [w138]
                stop <- w140 stop-if-true
                n54 = Increment(x=w138) -> (x+1=w137:i32)
                "AcqData" <- w137
                n55 = call "Get Image Data and Que.vi"("Acquisition count"=w137, "error in (no error)"=w144, "Exp params"=w135, "Refnum in"=w146, "Queue in"=w145) -> ("Logging Cluster"=w136:T20, "Session Out"=w133:T4, "Queue out"=w139:refnum<queue>)  [unwired: 4 in]
                n56 = Greater Or Equal?(x=w137, y=w142) -> (x >= y?=w141:bool)
                n57 = Or(x="StopAcq", y=w141) -> (x .or. y?=w140:bool)
              }
              n58 = property on="StopAcq" class="Bool"("DisabledEnum"=w122) -> ()  [unwired: 2 in, 2 out]
              n59 = call "Finish Time Series.vi"("Logging Cluster"=w123, "Session In"=w121, "Queue in"=w124) -> ()  [unwired: 9 in]
            }
            frame "Snapshot" {
              n60 = call "VarToData - TimeSeries.vi"("error in"=w155, "data"=w160) -> ("error out"=w154:errorcluster, "Exp params"=w149:T8)  [unwired: 3 in, 1 out]
              n61 = local read "Camera Controls"() -> (w156:T3)
              n62 = call "Preflight Time Series.vi"("error in"=w154, "Exp params"=w149, "Camera Controls"=w156) -> ("error out"=w157:errorcluster, "Exp params out"=w148:T8, "CamSession out"=w158:T4)  [unwired: 6 in]
              n63 = call "kernelTime.vi"("Action (Snap)"=Timer_actions."Total") -> ("Microseconds"=w153:u64)  [unwired: 9 in, 1 out]
              n64 = call "Get Image Data and Que.vi"("Acquisition count"=w153, "error in (no error)"=w157, "Exp params"=w148, "Refnum in"=w158, "Queue in"=w159) -> ("Logging Cluster"=w150:T20, "Session Out"=w147:T4, "Queue out"=w151:refnum<queue>)  [unwired: 4 in]
              n65 = call "Finish Time Series.vi"("Logging Cluster"=w150, "Session In"=w147, "Queue in"=w151) -> ()  [unwired: 9 in]
            }
            frame "Dynamic Time Series" {
              # "This will be for any experiements where we want to acquire images whilst simultaneously changing another param (laser power, hologram etc).\n\nIdeally we would only be acquiring data here and sending triggers to the hardware loop."
            }
          }
        }
        frame Error {
          w164 = u8[] []  # Image Data
          # "If this errors, the notif has been destroyed so we are shutting down.\n\nKill the que, and send true to the upper loop"
          n66 = Release Queue(queue=w166) -> ()  [unwired: 2 in, 3 out]
          n67 = Obtain Queue(name (unnamed)="Peak", element data type=w164) -> (queue out=w162:refnum<queue>)  [unwired: 3 in, 2 out]
          n68 = Release Queue(queue=w162, force destroy? (F)=TRUE) -> ()  [unwired: 1 in, 3 out]
        }
      }
    }
    n69 = while {
      tunnel: w51 -> [w81]
      tunnel: w53 -> [w77]
      tunnel: [w76] -> w49
      stop <- w76 stop-if-true
      # "Logging Child"
      n70 = Dequeue Element(queue=w77) -> (queue out=w78:refnum<queue>, element=w80:T20, error out=w79:errorcluster)  [unwired: 2 in, 1 out]
      n71 = case shown="No Error" w79 {
        selector: w79 -> [_ w100]
        tunnel: w81 -> [w86 w101]
        tunnel: [_ w100] -> w76
        tunnel: w80 -> [w84 _]
        tunnel: w78 -> [w82 _]
        frame No Error {
          n72 = Unbundle By Name(w84) -> ("Buffer Number"=→"Saving To Disk":i32, "Exp params.Save As"=w83:string)
          n73 = case shown="\"Finish Acquisition\"" w83 {
            tunnel: w86 -> [w88 _ _ _]
            tunnel: w84 -> [w87 w89 _ w99]
            tunnel: w82 -> [_ _ _ w97]
            frame "TIFF", Default {
              n74 = call "Save To TIFF.vi"("Logging Cluster"=w87, "img dst"=w88) -> ()  [unwired: 9 in, 1 out]
            }
            frame "TDMS" {
              n75 = call "Save to TDMS.vi"("Logging Cluster"=w89) -> ()  [unwired: 10 in, 1 out]
            }
            frame "RAW" {
            }
            frame "Finish Acquisition" {
              w93 = u8[] []  # Image Data
              w98 = T12."Enabled" ("Disabled")
              # "Restart Peak"
              # "Restart self"
              n76 = call "Finish Acquisition.vi"("Logging Cluster"=w99) -> ()  [unwired: 11 in]
              n77 = property on="Master Stop" class="Bool (strict)"("DisabledEnum"=w98) -> ()  [unwired: 2 in, 2 out]
              n78 = property on="Cam Live Display" class="Bool (strict)"("DisabledEnum"=w98) -> ()  [unwired: 2 in, 2 out]
              n79 = property on="Start Acquisition" class="Bool"("DisabledEnum"=w98) -> ()  [unwired: 2 in, 2 out]
              n80 = property on="StopAcq" class="Bool"("DisabledEnum"=w98) -> ()  [unwired: 2 in, 2 out]
              n81 = Release Queue(queue=w97) -> (error out=w91:errorcluster)  [unwired: 2 in, 2 out]
              n82 = Obtain Queue(name (unnamed)="Peak", element data type=w93, create if not found? (T)=FALSE, error in (no error)=w91) -> (queue out=w95:refnum<queue>, error out=w90:errorcluster)  [unwired: 1 in, 1 out]
              n83 = Release Queue(queue=w95, force destroy? (F)=TRUE, error in (no error)=w90) -> ()  [unwired: 3 out]
            }
          }
        }
        frame Error {
          n84 = call "IMAQ Dispose"("All Images? (No)"=FALSE, "Image"=w101) -> ()  [unwired: 4 in, 1 out]
        }
      }
    }
    n85 = timed-loop {
      tunnel: w44 -> [w61]
      tunnel: w41 -> [w58]
      tunnel: [w57] -> w40
      timing: w39 -> [_]
      timing-out: [_] -> w38
      stop <- w57 stop-if-true
      # "Peaking Child"
      n86 = node-c288() -> ()  [unwired: 1 in]
      n87 = Dequeue Element(queue=w61) -> (element=w59:u8[], error out=w60:errorcluster)  [unwired: 2 in, 2 out]
      n88 = case shown="Error .." w60 {
        selector: w60 -> [_ w73]
        tunnel: w59 -> [w68 _]
        tunnel: w58 -> [w67 w71]
        tunnel: [_ w73] -> w57
        frame No Error {
          n89 = global read "Global Controls.vi" "Camera Controls"() -> (w66:T3)
          n90 = Unbundle By Name(w66) -> ("Camera ROI.Height"=w65:u32, "Camera ROI.Width"=w64:u32)
          n91 = Reshape Array(w68, w65, w64) -> (w69:u8[][])
          n92 = call "IMAQ ArrayToImage"("Image Pixels (U8)"=w69, "Image"=w67) -> ("Image Out"=w70:T1)  [unwired: 8 in, 1 out]
          n93 = local write "xiCam"(w70) -> ()
        }
        frame Error {
          n94 = call "IMAQ Dispose"("All Images? (No)"=FALSE, "Image"=w71) -> ()  [unwired: 4 in, 1 out]
        }
      }
      n95 = node-c288() -> ()  [unwired: 1 out]
    }
    n96 = node-c288(w38) -> ()  [unwired: 1 out]
    n97 = Compound Arithmetic op=AND(w48, w49, w40) -> (w50:bool)
  }
  n98 = timed-loop {
    tunnel: w16 -> [w167]
    timing: w3 -> [_]
    timing-out: [_] -> w2
    stop <- w169 stop-if-true
    # "User Interface MASTER"
    n99 = node-c288() -> ()  [unwired: 1 in]
    n100 = event shown="[13] \"Spots.Spot Params\", \"Zernikes\", \"SLM Parameters\": Value Change" {
      selector: _ -> [_ _ _ _ _ _ _ _ _ _ _ _ _ _ _ _ _ _ _]
      dyn-events: _ -> [_ _ _ _ _ _ _ _ _ _ _ _ _ _ _ _ _ _ _]
      timeout: 100 -> [_ _ _ _ _ _ _ _ _ _ _ _ _ _ _ _ _ _ _]
      tunnel: [_ _ _ _ _ _ _ _ _ _ _ _ _ _ _ _ _ _ TRUE] -> w169
      tunnel: w167 -> [_ w187 _ w196 _ _ _ _ w216 w227 w262 w292 _ w328 _ _ _ _ w375]
      event Timeout {
        # "Be carefull when adding things here. If you need a critical global to be updating before it is picked up else where, this is not the place , as we have no assurance that a race condition will not occur."
        n101 = event-data() -> ()  [unwired: 1 in, 1 out]
        n102 = global read "Global Controls.vi" "SLM Params"() -> (w176:T11)
        n103 = First Call?() -> (First Call?: T/F=w173:bool)
        n104 = case shown="False" w173 {
          selector: w173 -> [_ w178]
          frame False {
          }
          frame True {
            "READY" <- w178
          }
        }
        n105 = Unbundle By Name(w176) -> ("Board ID"=w177:i32)
        n106 = global write "Global Controls.vi" "Camera Controls"("Camera Controls") -> ()
        n107 = global write "Global Controls.vi" "SLM to IMAQ"("SLM to IMAQ") -> ()
        n108 = call <userlib>:"Read SLM temperature.vi"("board IN"=w177) -> ("temperature"=→"SLM Temp (C)":dbl)  [unwired: 8 in, 2 out]
      }
      event "Cam Live Display": Value Change {
        w184 = T12."Disabled and Grayed Out" ("Disabled")
        n109 = event-data() -> ()  [unwired: 1 in, 1 out]
        n110 = local read "Camera Controls"() -> (w182:T3)
        n111 = Unbundle By Name(w187) -> ("Live Display"=w186:refnum<notifier>)
        n112 = To Variant(anything=w182) -> (Variant=w183:variant)
        n113 = call "FormatNotification.vi"("Param in variant form"=w183, "message"="LiveCam") -> ("Notification"=w180:variant)  [unwired: 2 in]
        n114 = property on="stop live" class="Bool (strict)"("DisabledEnum"=T12."Enabled" ("Disabled")) -> ()  [unwired: 2 in, 2 out]
        n115 = Send Notification(notification=w180, notifier=w186) -> ()  [unwired: 1 in, 2 out]
        n116 = property on="Master Stop" class="Bool (strict)"("DisabledEnum"=w184) -> ()  [unwired: 2 in, 2 out]
        n117 = property on="Start Acquisition" class="Bool"("DisabledEnum"=w184) -> ()  [unwired: 2 in, 2 out]
        n118 = property on="Cam Live Display" class="Bool (strict)"("DisabledEnum"=w184, "Value"=FALSE ("Cam Live Display")) -> ()  [unwired: 2 in, 2 out]
      }
      event "stop live": Value Change {
        w189 = T12."Enabled" ("Disabled")
        n119 = event-data() -> ()  [unwired: 1 in, 1 out]
        n120 = property on="stop live" class="Bool (strict)"("DisabledEnum"=T12."Disabled and Grayed Out" ("Disabled")) -> ()  [unwired: 2 in, 2 out]
        n121 = property on="Master Stop" class="Bool (strict)"("DisabledEnum"=w189) -> ()  [unwired: 2 in, 2 out]
        n122 = property on="Cam Live Display" class="Bool (strict)"("DisabledEnum"=w189) -> ()  [unwired: 2 in, 2 out]
        n123 = property on="Start Acquisition" class="Bool"("DisabledEnum"=w189) -> ()  [unwired: 2 in, 2 out]
      }
      event "Start Acquisition": Value Change {
        w195 = T12."Disabled and Grayed Out" ("Disabled")
        n124 = event-data() -> ()  [unwired: 1 in, 1 out]
        n125 = Unbundle By Name(w196) -> ("Acquisition"=w197:refnum<notifier>)
        n126 = call "Check if Folder exists.vi"("Exp Params in"="Exp Params") -> ("Exp Params out"=w193:T8)  [unwired: 9 in, 1 out]
        n127 = Unbundle By Name(w193) -> ("Experiment Type"=w192:string)
        n128 = To Variant(anything=w193) -> (Variant=w194:variant)
        n129 = call "FormatNotification.vi"("Param in variant form"=w194, "message"=w192) -> ("Notification"=w191:variant)  [unwired: 2 in]
        n130 = Send Notification(notification=w191, notifier=w197) -> ()  [unwired: 1 in, 2 out]
        n131 = property on="Cam Live Display" class="Bool (strict)"("DisabledEnum"=w195) -> ()  [unwired: 2 in, 2 out]
        n132 = property on="Master Stop" class="Bool (strict)"("DisabledEnum"=w195) -> ()  [unwired: 2 in, 2 out]
        n133 = property on="Start Acquisition" class="Bool"("DisabledEnum"=w195) -> ()  [unwired: 2 in, 2 out]
      }
      event "AcquireSnap": Value Change {
        n134 = event-data() -> ("NewVal"=w201:bool)  [unwired: 1 in]
        n135 = Not(x=w201) -> (.not. x?=w200:bool)
        n136 = property on="stop live" class="Bool (strict)"("Val(Sgnl)"=w200) -> (error out=w199:errorcluster)  [unwired: 2 in, 1 out]
        n137 = property on="Exp Params" class="Clust (strict)"(error in=w199) -> (error out=w198:errorcluster, "Value"=w204:T8)  [unwired: 1 in, 1 out]
        n138 = Bundle By Name(cluster=w204, "Experiment Type"="Snapshot") -> (w205:T8)
        n139 = property on="Exp Params" class="Clust (strict)"(error in=w198, "Val(Sgnl)"=w205) -> (error out=w202:errorcluster)  [unwired: 1 in, 1 out]
        n140 = property on="Start Acquisition" class="Bool"(error in=w202, "Val(Sgnl)"=w201) -> ()  [unwired: 1 in, 2 out]
      }
      event Value Change {
        n141 = event-data() -> ("NewVal"=w207:i32)  [unwired: 1 in]
        n142 = To Double Precision Float(number=w207) -> (double precision float=w206:dbl)
        n143 = property on="Saving To Disk" class="Slide (strict)"("Scale.Maximum"=w206) -> ()  [unwired: 2 in, 2 out]
        n144 = property on="AcqData" class="Slide (strict)"("Scale.Maximum"=w206) -> ()  [unwired: 2 in, 2 out]
      }
      event Value Change {
        n145 = event-data() -> ("NewVal"=w208:string)  [unwired: 1 in]
        n146 = case shown="\"False\", Default" w208 {
          frame "False", Default {
          }
          frame "Snapshot" {
            n147 = property on="Streaming" class="Bool (strict)"("Value"=TRUE) -> ()  [unwired: 2 in, 2 out]
            n148 = property on="TSFrames" class="DigNum (strict)"("Value"=1) -> ()  [unwired: 2 in, 2 out]
            n149 = property on="Save As" class="CmbBox"("Value"="TIFF") -> ()  [unwired: 2 in, 2 out]
          }
        }
      }
      event Value Change {
        n150 = event-data() -> ("NewVal"=w213:bool)  [unwired: 1 in]
        n151 = Not(x=w213) -> (.not. x?=w212:bool)
        n152 = property on="TSfps" class="DigNum (strict)"("Visible"=w212) -> ()  [unwired: 2 in, 2 out]
      }
      event Value Change {
        n153 = event-data() -> ()  [unwired: 1 in, 1 out]
        n154 = Unbundle By Name(w216) -> ("Instrument Control"=w217:refnum<notifier>)
        n155 = To Variant(anything="Ventus Controls") -> (Variant=w215:variant)
        n156 = call "FormatNotification.vi"("Param in variant form"=w215, "message"="Update Ventus") -> ("Notification"=w218:variant)  [unwired: 2 in]
        n157 = Send Notification(notification=w218, notifier=w217) -> ()  [unwired: 1 in, 2 out]
      }
      event Value Change {
        n158 = event-data() -> ("OldVal"=w243:T3, "NewVal"=w242:T3)  [unwired: 1 in]
        n159 = Not Equal?(x=w243, y=w242) -> (x != y?=w241:T23)
        n160 = Unbundle By Name(w241) -> ("Exposure Time (ms)"=w222:bool, "Camera ROI.Width"=w240:bool, "Camera ROI.Height"=w239:bool, "Camera ROI.Offset X"=w238:bool, "Camera ROI.Offset Y"=w237:bool)
        n161 = property on="LIVE" class="Bool (strict)"() -> ("Value"=w223:bool)  [unwired: 2 in, 2 out]
        n162 = Not(x=w222) -> (.not. x?=w221:bool)
        n163 = Build Array(w222, w240, w239, w238, w237) -> (w236:bool[])
        n164 = And(x=w223, y=w221) -> (x .and. y?=w224:bool)
        n165 = Search 1D Array(1D array=w236, element=TRUE) -> (index of element=w234:i32)  [unwired: 1 in]
        n166 = case shown="True" w224 {
          selector: w224 -> [_ w246]
          tunnel: w227 -> [w245 w247]
          tunnel: [w245 w247] -> w226
          frame False {
          }
          frame True {
            n167 = flat-sequence {
              tunnel: w246 -> [w248]
              frame #0 {
                n168 = property on="stop live" class="Bool (strict)"("Val(Sgnl)"=w248) -> ()  [unwired: 2 in, 2 out]
              }
              frame #1 {
                n169 = Wait (ms)(milliseconds to wait=u32 100) -> ()  [unwired: 1 out]
              }
            }
          }
        }
        n170 = local read "Camera Controls"() -> (w220:T3)
        n171 = case shown="0, Default" w234 {
          tunnel: ["ExposureTime" "Width" "Height" "OffsetX" "OffsetY"] -> w228
          frame 0, Default {
          }
          frame 1 {
          }
          frame 2 {
          }
          frame 3 {
          }
          frame 4 {
          }
        }
        n172 = Bundle By Name(cluster=w220, "Command"=w228) -> (w229:T3)
        n173 = Unbundle By Name(w226) -> ("Instrument Control"=w233:refnum<notifier>)
        n174 = To Variant(anything=w229) -> (Variant=w232:variant)
        n175 = call "FormatNotification.vi"("Param in variant form"=w232, "message"="Update Cam") -> ("Notification"=w230:variant)  [unwired: 2 in]
        n176 = Send Notification(notification=w230, notifier=w233) -> (error out=w225:errorcluster)  [unwired: 1 in, 1 out]
        n177 = case shown="True" w224 {
          selector: w224 -> [_ w244]
          tunnel: w225 -> [_ _]
          frame False {
          }
          frame True {
            n178 = property on="Cam Live Display" class="Bool (strict)"("Val(Sgnl)"=w244) -> ()  [unwired: 2 in, 2 out]
          }
        }
      }
      event "Reset ROI": Value Change {
        n179 = event-data() -> ()  [unwired: 1 in, 1 out]
        n180 = property on="LIVE" class="Bool (strict)"() -> ("Value"=w259:bool)  [unwired: 2 in, 2 out]
        n181 = local read "Camera Controls"() -> (w257:T3)
        n182 = Bundle By Name(cluster=w257, "Camera ROI"=T22 {"Width"=2048, "Height"=2048, "Offset X"=0, "Offset Y"=0}) -> (w255:T3)
        n183 = case shown="True" w259 {
          selector: w259 -> [_ w280]
          tunnel: w262 -> [w279 w281]
          tunnel: [w279 w281] -> w261
          frame False {
          }
          frame True {
            n184 = flat-sequence {
              tunnel: w280 -> [w282]
              frame #0 {
                n185 = property on="stop live" class="Bool (strict)"("Val(Sgnl)"=w282) -> ()  [unwired: 2 in, 2 out]
              }
              frame #1 {
                n186 = Wait (ms)(milliseconds to wait=u32 100) -> ()  [unwired: 1 out]
              }
            }
          }
        }
        n187 = property on="Camera Controls" class="Clust (strict)"("Value"=w255) -> ()  [unwired: 2 in, 2 out]
        n188 = for {
          N: 4 -> [_]
          tunnel: w261 -> [w268]
          tunnel: [w267] -> w260
          tunnel: w255 -> [w265]
          i -> [w264]
          n189 = case shown="0, Default" w264 {
            tunnel: ["OffsetX" "OffsetY" "Width" "Height"] -> w269
            frame 0, Default {
            }
            frame 1 {
            }
            frame 2 {
            }
            frame 3 {
            }
          }
          n190 = Bundle By Name(cluster=w265, "Command"=w269) -> (w266:T3)
          n191 = Unbundle By Name(w268) -> ("Instrument Control"=w273:refnum<notifier>)
          n192 = To Variant(anything=w266) -> (Variant=w272:variant)
          n193 = call "FormatNotification.vi"("Param in variant form"=w272, "message"="Update Cam") -> ("Notification"=w270:variant)  [unwired: 2 in]
          n194 = Wait (ms)(milliseconds to wait=u32 20) -> ()  [unwired: 1 out]
          n195 = Send Notification(notification=w270, notifier=w273) -> (error out=w267:errorcluster)  [unwired: 1 in, 1 out]
        }
        n196 = case shown="True" w259 {
          selector: w259 -> [_ w278]
          tunnel: w260 -> [_ _]
          frame False {
          }
          frame True {
            n197 = property on="Cam Live Display" class="Bool (strict)"("Val(Sgnl)"=w278) -> ()  [unwired: 2 in, 2 out]
          }
        }
      }
      event "Set ROI": Value Change {
        n198 = event-data() -> ()  [unwired: 1 in, 1 out]
        n199 = property on="LIVE" class="Bool (strict)"() -> ("Value"=w289:bool)  [unwired: 2 in, 2 out]
        n200 = property on="xiCam" class="ImageControl"() -> ("ROI"=w285:T24)  [unwired: 2 in, 2 out]
        n201 = call "Convert ROI.vi"("ROI"=w285) -> ("Camera ROI"=w284:T22)
        n202 = case shown="True" w289 {
          selector: w289 -> [_ w310]
          tunnel: w292 -> [w309 w311]
          tunnel: [w309 w311] -> w291
          frame False {
          }
          frame True {
            n203 = flat-sequence {
              tunnel: w310 -> [w312]
              frame #0 {
                n204 = property on="stop live" class="Bool (strict)"("Val(Sgnl)"=w312) -> ()  [unwired: 2 in, 2 out]
              }
              frame #1 {
                n205 = Wait (ms)(milliseconds to wait=u32 100) -> ()  [unwired: 1 out]
              }
            }
          }
        }
        n206 = local read "Camera Controls"() -> (w287:T3)
        n207 = Bundle By Name(cluster=w287, "Camera ROI"=w284) -> (w286:T3)
        n208 = for {
          N: 4 -> [_]
          tunnel: w291 -> [w298]
          tunnel: [w297] -> w290
          tunnel: w286 -> [w295]
          i -> [w294]
          n209 = case shown="1" w294 {
            tunnel: ["Height" "Width" "OffsetY" "OffsetX"] -> w299
            frame 0, Default {
            }
            frame 1 {
            }
            frame 2 {
            }
            frame 3 {
            }
          }
          n210 = Bundle By Name(cluster=w295, "Command"=w299) -> (w296:T3)
          n211 = Unbundle By Name(w298) -> ("Instrument Control"=w303:refnum<notifier>)
          n212 = To Variant(anything=w296) -> (Variant=w302:variant)
          n213 = call "FormatNotification.vi"("Param in variant form"=w302, "message"="Update Cam") -> ("Notification"=w300:variant)  [unwired: 2 in]
          n214 = Wait (ms)(milliseconds to wait=u32 20) -> ()  [unwired: 1 out]
          n215 = Send Notification(notification=w300, notifier=w303) -> (error out=w297:errorcluster)  [unwired: 1 in, 1 out]
        }
        n216 = property on="Camera Controls" class="Clust (strict)"("Value"=w286) -> ()  [unwired: 2 in, 2 out]
        n217 = case shown="True" w289 {
          selector: w289 -> [_ w308]
          tunnel: w290 -> [_ _]
          frame False {
          }
          frame True {
            n218 = property on="Cam Live Display" class="Bool (strict)"("Val(Sgnl)"=w308) -> ()  [unwired: 2 in, 2 out]
          }
        }
      }
      event Value Change {
        # "Generate 9 by 9 grid of spots with a noise factor to stop negative order overlap"
        n219 = event-data() -> ()  [unwired: 1 in, 1 out]
        n220 = call "9by9GridOfSpots.vi"("GridSpotsNoiseAmp"="GridSpotsNoiseAmp", "Grid Size Y"="Grid Size Y", "Grid Size x"="Grid Size x") -> ("Spot Params"=w314:T6)  [unwired: 8 in]
        n221 = local read "Spots"() -> (w316:T5)
        n222 = Bundle By Name(cluster=w316, "Spot Params"=w314) -> (w315:T5)
        n223 = property on="Spots" class="Clust (strict)"("Val(Sgnl)"=w315) -> ()  [unwired: 2 in, 2 out]
      }
      event Value Change {
        n224 = event-data() -> ()  [unwired: 1 in, 6 out]
        n225 = Unbundle By Name(w328) -> ("Instrument Control"=w327:refnum<notifier>)
        n226 = global write "Global Controls.vi" "Spots"("Spots") -> ()
        n227 = global write "Global Controls.vi" "SLM Params"("SLM Parameters") -> ()
        n228 = Bundle("Spots"="Spots", "SLM Parameters"="SLM Parameters", "Zernikes"="Zernikes") -> (w321:T25)  [unwired: 1 in]
        n229 = To Variant(anything=w321) -> (Variant=w320:variant)
        n230 = call "FormatNotification.vi"("Param in variant form"=w320, "message"="Update SLM") -> ("Notification"=w322:variant)  [unwired: 2 in]
        n231 = Send Notification(notification=w322, notifier=w327) -> ()  [unwired: 1 in, 2 out]
      }
      event "LUT Graph": Cursor Move {
        # "Generate LUT from cursor position, then save new LUT to disk, then load LUT to SLM"
        n232 = event-data() -> ()  [unwired: 1 in, 1 out]
        n233 = local read "SLM Parameters"() -> (w333:T11)
        n234 = property on="LUT Graph" class="XYGraph (strict)"() -> ("CrsrList"=w335:T26)  [unwired: 2 in, 2 out]
        n235 = for {
          tunnel: w335 -> [w338] mode=indexing
          tunnel: [w337] -> w336 mode=indexing
          n236 = Unbundle By Name(w338) -> ("Position"=w337:cluster{"X":dbl, "Y":dbl})
        }
        n237 = Unbundle By Name(w333) -> ("Board ID"=w332:i32)
        n238 = call "setPhaseBlazingTable.vi"("Anchor Points"=w336) -> ("blazing graph"=→"LUT Graph":cluster{dbl, dbl}[], "blazing table"=w331:dbl[])  [unwired: 2 in]
        n239 = call "Save LUT to Disk.vi"("file (use dialog)"=path "D:/Software/Optical-Prime/Instruments/SLM/LUT.lut", "Blaze Data"=w331) -> ("file (use dialog) out"=w334:path)  [unwired: 9 in]
        n240 = call <userlib>:"Load LUT file.vi"("LUT_file"=w334, "board IN"=w332) -> ()  [unwired: 7 in, 3 out]
      }
      event "SaveCurrentXML": Value Change {
        n241 = event-data() -> ()  [unwired: 1 in, 1 out]
        n242 = call "Write Settings XML.vi"() -> ("error out"=w340:errorcluster, "XML File Path(duplicate)"=w344:path)  [unwired: 10 in]
        n243 = Strip Path(path=w344) -> (name=w342:string)  [unwired: 1 out]
        n244 = Concatenate Strings("Settings saved to ", w342) -> (w341:string)
        n245 = case shown="No Error" w340 {
          tunnel: w341 -> [w346 _]
          tunnel: [FALSE ("SaveCurrentXML") FALSE ("SaveCurrentXML")] -> w339
          frame No Error {
            n246 = call "Settings Saved"("Message"=w346) -> ()  [unwired: 9 in, 2 out]
          }
          frame Error {
            n247 = call "Save Failed"() -> ()  [unwired: 10 in, 2 out]
          }
        }
        n248 = property on="SaveCurrentXML" class="Bool (strict)"("Value"=w339) -> ()  [unwired: 2 in, 2 out]
      }
      event "LoadXML": Value Change {
        n249 = event-data() -> ()  [unwired: 1 in, 1 out]
        n250 = local read "Camera Controls"() -> (w361:T3)
        n251 = local read "Ventus Controls"() -> (w360:T7)
        n252 = global read "Global Controls.vi" "SLM Params"() -> (w362:T11)
        n253 = Unbundle By Name(w362) -> ("Board ID"=w358:i32)
        n254 = Unbundle By Name(w361) -> ("cam0 Session"=w357:T4)
        n255 = Unbundle By Name(w360) -> ("VISA Refnum"=w356:refnum<visa-resource-name>)
        n256 = call "Read in XML.vi"("Path to XML"=path "") -> ("error out"=w363:errorcluster, "OpticalPrime Ctrls For Saving"=w359:T15)  [unwired: 9 in]
        n257 = Bundle By Name(cluster=w359, "SLM Parameters.Board ID"=w358, "Camera Controls.cam0 Session"=w357, "Ventus Controls.VISA Refnum"=w356) -> (w355:T15)
        n258 = call "Push All Ctrls.vi"("error in"=w363, "OpticalPrime Ctrls For Saving"=w355) -> ("error out"=w349:errorcluster, "OpticalPrime Ctrls For Saving out"=w353:T15)  [unwired: 8 in]
        n259 = Unbundle By Name(w353) -> ("Ventus Controls"=w351:T7, "Camera Controls"=w352:T3, "SLM Parameters"=w350:T11)
        n260 = local write "Camera Controls"(w352) -> ()
        n261 = global write "Global Controls.vi" "SLM Params"(w350) -> ()
        n262 = local write "Ventus Controls"(w351) -> ()
        n263 = property on="LoadXML" class="Bool (strict)"(error in=w349, "Value"=FALSE ("LoadXML")) -> ()  [unwired: 1 in, 2 out]
      }
      event "Show Hologram": Value Change {
        n264 = event-data() -> ()  [unwired: 1 in, 1 out]
        n265 = call "Display Hologram.vi"() -> ()  [unwired: 1 out]
      }
      event "Master Stop": Value Change {
        n266 = event-data() -> ()  [unwired: 1 in, 1 out]
        n267 = Unbundle By Name(w375) -> ("Acquisition"=w371:refnum<notifier>, "Instrument Control"=w374:refnum<notifier>, "Live Display"=w373:refnum<notifier>)
        n268 = local read "Camera Controls"() -> (w377:T3)
        n269 = local read "SLM Parameters"() -> (w368:T11)
        n270 = Unbundle By Name(w377) -> ("cam0 Session"=w376:T4)
        n271 = Release Notifier(notifier=w373) -> (error out=w370:errorcluster)  [unwired: 2 in, 2 out]
        n272 = Release Notifier(notifier=w374, error in (no error)=w370) -> (error out=w372:errorcluster)  [unwired: 1 in, 2 out]
        n273 = Release Notifier(notifier=w371, error in (no error)=w372) -> (error out=w367:errorcluster)  [unwired: 1 in, 2 out]
        n274 = call "ShutDown SLM.vi"("error in (no error)"=w367, "SLM Parameters"=w368) -> ("error out"=w366:errorcluster)  [unwired: 9 in]
        n275 = call <vilib>:"IMAQdx Close Camera.vi"("error in"=w366, "Session In"=w376) -> ("error out"=w365:errorcluster)  [unwired: 9 in]
        n276 = call "Write Settings XML.vi"("error in (no error)"=w365, "path"=path "E:/Software/Optical-Prime/_Last Session Settings.xml") -> ("error out"=w364:errorcluster)  [unwired: 8 in, 1 out]
        n277 = call <vilib>:"Clear Errors.vi"("error in (no error)"=w364) -> ()  [unwired: 5 in, 2 out]
      }
    }
    n278 = node-c288() -> ()  [unwired: 1 out]
  }
  n279 = while {
    tunnel: w16 -> [w380]
    tunnel: w20 -> [w383]
    stop <- w385 stop-if-true
    # "Live Camera Display"
    n280 = Unbundle By Name(w380) -> ("Live Display"=w379:refnum<notifier>)
    n281 = Wait on Notification(notifier=w379) -> (notifier out=w381:refnum<notifier>, notification=w382:variant, error out=w384:errorcluster)  [unwired: 3 in, 1 out]
    n282 = case shown="No Error" w384 {
      tunnel: [_ TRUE] -> w385
      tunnel: w383 -> [w397 w412]
      tunnel: w382 -> [w396 _]
      tunnel: w381 -> [_ _]
      frame No Error {
        n283 = Variant To Data(type=T27 {"message"="", "data"=variant}, Variant=w396) -> (data=w394:T27)  [unwired: 1 in, 1 out]
        n284 = Unbundle By Name(w394) -> ("data"=w393:variant)
        n285 = Variant To Data(type=T3 {"Exposure Time (ms)"=0, "cam0 Session"="cam0", "Camera ROI"={"Width"=0, "Height"=0, "Offset X"=0, "Offset Y"=0}, "Command"=""} ("Camera Controls"), Variant=w393) -> (data=w388:T3)  [unwired: 1 in, 1 out]
        n286 = call "Preflight Time Series.vi"("Camera Controls"=w388) -> ("error out"=w391:errorcluster, "CamSession out"=w390:T4)  [unwired: 8 in, 1 out]
        n287 = while {
          tunnel: w391 -> [w408]
          shift-right: [w405] -> _
          shift-left: u64[] [] -> [w406]
          tunnel: [FALSE] -> w386
          tunnel: w397 -> [w404]
          shift-right: [w401] -> w387
          shift-left: w390 -> [w402]
          stop <- "stop live" stop-if-true
          n288 = call "Live view.vi"("Timings Array"=w406, "error in (no error)"=w408, "dst image"=w404, "CamSession in"=w402) -> ("Frame Rate (Hz)"=→"fps":dbl, "Image out"=→"xiCam":T1, "CamSession Out"=w401:T4, "Image Saturated"=w400:bool, "Timings Array out"=w405:u64[], "ImgHist"=→"ImgHist":u32[])  [unwired: 1 in, 1 out]
          "ImgSat" <- w400
          n289 = property on="ImgSat" class="Bool (strict)"("Visible"=w400) -> ()  [unwired: 2 in, 2 out]
          "LIVE" <- TRUE ("LIVE")
        }
        n290 = call <vilib>:"IMAQdx Unconfigure Acquisition.vi"("Session In"=w387) -> ()  [unwired: 9 in, 2 out]
        n291 = property on="stop live" class="Bool (strict)"("Value"=w386) -> ()  [unwired: 2 in, 2 out]
        n292 = property on="LIVE" class="Bool (strict)"("Value"=w386) -> ()  [unwired: 2 in, 2 out]
      }
      frame Error {
        n293 = call "IMAQ Dispose"("All Images? (No)"=FALSE, "Image"=w412) -> ()  [unwired: 4 in, 1 out]
      }
    }
  }
  n294 = while {
    tunnel: w16 -> [w415]
    stop <- w418 stop-if-true
    # "Just comms with SDKs and hardware. Avoid adding any processing or conditionals here. Instead add thes in either UI parent or Acquisition child and message back to here"
    # "Hardware control Child"
    n295 = Unbundle By Name(w415) -> ("Instrument Control"=w414:refnum<notifier>)
    n296 = Wait on Notification(notifier=w414) -> (notifier out=w416:refnum<notifier>, notification=w417:variant, error out=w419:errorcluster)  [unwired: 3 in, 1 out]
    n297 = case shown="No Error" w419 {
      tunnel: [_ TRUE] -> w418
      tunnel: w417 -> [w424 _]
      tunnel: w416 -> [w422 _]
      frame No Error {
        n298 = call "Receive notification.vi"("Variant"=w424, "notifier in"=w422) -> ("message"=w420:string, "data"=w423:variant, "notifier out"=w421:refnum<notifier>)  [unwired: 6 in, 1 out]
        n299 = case shown="\"Update SLM\"" w420 {
          tunnel: w423 -> [w428 w431 w435]
          tunnel: w421 -> [_ _ _]
          frame "Update Cam", Default {
            n300 = call "VarToData - Live.vi"("data"=w428) -> ("param"=w425:u32, "Command"=w427:string, "cam0 Session"=w426:T4)  [unwired: 8 in]
            n301 = property class="IMAQdx"(reference=w426, "ActiveAttribute"=w427, "ValueU32"=w425) -> ()  [unwired: 1 in, 2 out]
          }
          frame "Update SLM" {
            n302 = Variant To Data(type=T25 {"Spots"={"Spot Params"=[], "Add Spot"=FALSE, "Remove Spot"=FALSE, "Clear All Spots"=FALSE, "Save Spots"=FALSE, "Generate Spots"=FALSE, "Generate Spot Pattern"=""}, "SLM Parameters"={"Width"=0.0, "Height"=0.0, "Board ID"=0, "Centre Y"=0.0, "Centre X"=0.0}, "Zernikes"={"enabled"=FALSE, "AstigX"=0.0, "AstigY"=0.0, "ComaX"=0.0, "ComaY"=0.0, "SecAstigX"=0.0, "SecAstigY"=0.0, "SecComaX"=0.0, "SecComaY"=0.0}} ("All SLM"), Variant=w431) -> (data=w430:T25)  [unwired: 1 in, 1 out]
            n303 = call "PCIe SLM - Calculate Image.vi"("Spots, Params and Zernike"=w430) -> ()  [unwired: 10 in, 1 out]
          }
          frame "Update Ventus" {
            n304 = Variant To Data(type=T7 {"Ventus Power"=0.0, "Open Serial"=FALSE, "VISA Refnum"=""} ("Manlight Controls"), Variant=w435) -> (data=w434:T7)  [unwired: 1 in, 1 out]
            n305 = Unbundle By Name(w434) -> ("VISA Refnum"=w433:refnum<visa-resource-name>, "Ventus Power"=w432:dbl)
            n306 = call "Ventus - Update Power.vi"("Power (%)"=w432, "VISA resource name"=w433) -> ()  [unwired: 4 in, 2 out]
          }
        }
      }
      frame Error {
      }
    }
  }
  n307 = node-c288(w2) -> ()
  n308 = disable-structure shown="Enabled" {
    frame Disabled {
      n309 = property class="IMAQdx"("ActiveAttribute"="Height", "ValueU32"=u32 200) -> ()  [unwired: 2 in, 2 out]
    }
    frame Enabled {
    }
  }
